vi "WLAN - RxMeasure - Test  - Readwaveform.vi"(0 "VSG Resource Name":refnum<k15>="rio0", 1 "Idle Time/s (With Ack)":dbl, 5 "file path":path, 7 "Power Level(dBm)":dbl, 9 "numPackets":i32=200, 11 "Carrier Frequency(Hz)":dbl, 12 "Path Loss":dbl=1.0) -> ()   [LabVIEW 2010]
uses:
  <instrlib>/niRFSG/niRFSG.llb/niRFSG Ref Clock Sources.ctl
panel:
  in  "stop":bool
  out "LoopTime/ms":u32
  in  "Tab Control":enum32{"Rx_Test Settings", "HW "}(tab)=enum."HW "
  in  "error in (no error)":errorcluster
  out "error out":errorcluster
  # "GET PACKET COUNT (1)"
  # "PACKET STOP"
  # "PACKET START"
  # "GET PACKET COUNT (2)"
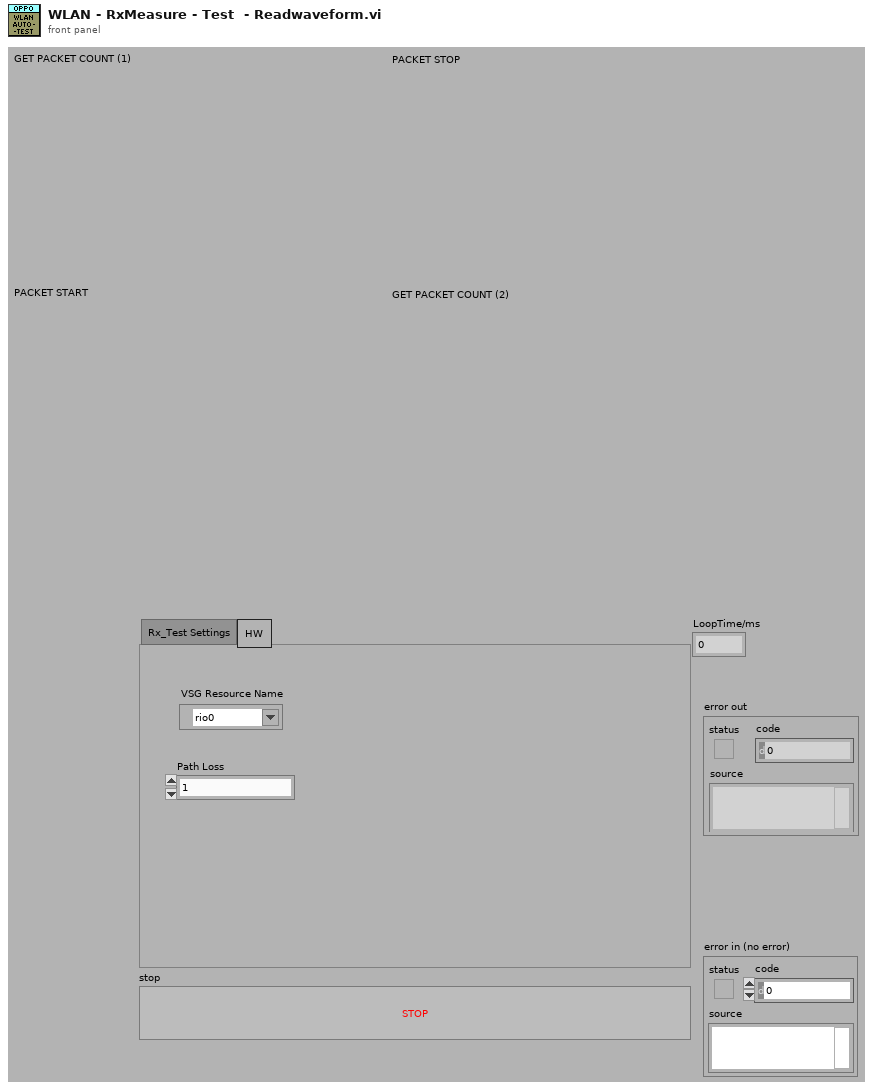
[diagram p1: front panel]
types:
  T1 = typedef "niRFSG Ref Clock Sources.ctl" = string
  T2 = typedef "WLAN - TV - RW - INC - RxTestParameters.ctl" = cluster{"wfm Size in msec":i32, "actual headroom (dB)":dbl, "Size in Samples":i32[], "40M?":bool, "Standard ":i32, "wfm size sec (dbl)":dbl, "dt":dbl, "Channel Bandwidth (Hz)":dbl, "Payload Data Length (bytes)":i32, "80211n PLCP Frame Format":i32, "DSSS Data Rate (Mbps)":i32, "OFDM Data Rate (Mbps)":i32, "MCS Index":i32, "Fc(Hz)":dbl, "#Packets":i32}
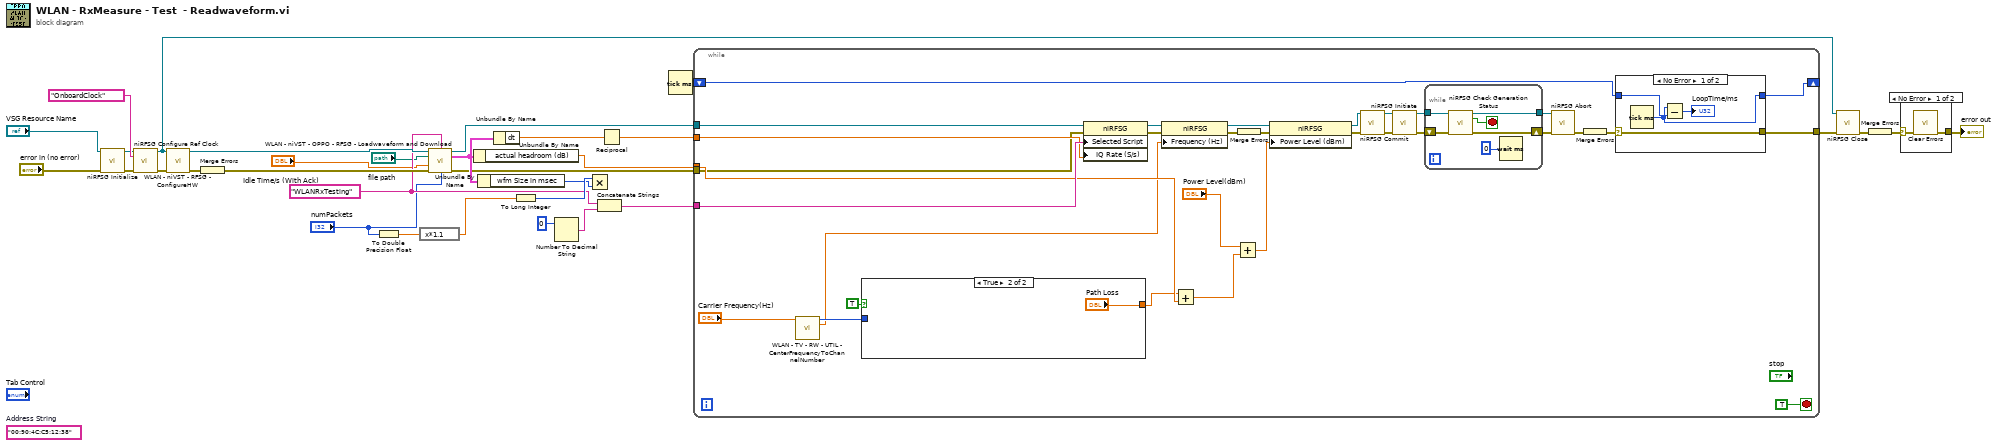
[diagram p0: block diagram]
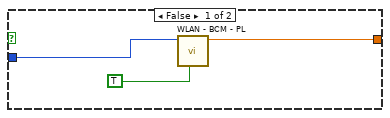
[diagram p2: hidden frame]
diagram:
  w14 = "WLANRxTesting" ("Arb:Selected Script")
  (unwired) "00:90:4C:C5:12:38"  # Address String
  n1 = call <instrlib>:"niRFSG Initialize.vi"("resource name"="VSG Resource Name", "error in"="error in (no error)") -> ("instrument handle"=w20:refnum<k15>, "error out"=w22:errorcluster)  [unwired: 12 in]
  n2 = call <instrlib>:"niRFSG Configure Ref Clock.vi"("instrument handle"=w20, "ref clock source"=T1 "OnboardClock", "error in"=w22) -> ("instrument handle out"=w23:refnum<k15>, "error out"=w21:errorcluster)  [unwired: 11 out]
  n3 = call "WLAN - niVST - RFSG - ConfigureHW.vi"("instrument handle"=w23, "error in"=w21) -> ("instrument handle"=w28:refnum<k15>, "error out"=w27:errorcluster)  [unwired: 12 in]
  n4 = Merge Errors(w27) -> (w15:errorcluster)
  n5 = To Double Precision Float(number="numPackets") -> (double precision float=w18:dbl)
  n6 = expression code="x*1.1"(w18) -> (w19:dbl)
  n7 = call "WLAN - niVST - OPPO - RFSG - Loadwaveform and Download.vi"("instrument handle"=w28, "ScriptName<index>"=w14, "file path"="file path", "Idle Time (With Ack)"="Idle Time/s (With Ack)", "error in"=w15, "numPackets"="numPackets") -> ("instrument handle"=w3:refnum<k15>, "Rx_Test Parameters"=w16:T2, "error out"=w4:errorcluster)  [unwired: 7 in]
  n8 = Unbundle By Name(w16) -> ("actual headroom (dB)"=w8:dbl)
  n9 = Unbundle By Name(w16) -> ("wfm Size in msec"=w9:i32)
  n10 = Unbundle By Name(w16) -> ("dt"=w10:dbl)
  n11 = To Long Integer(number=w19) -> (32bit integer=w17:i32)
  n12 = Number To Decimal String(number=0) -> (decimal integer string=w13:string)  [unwired: 1 in]
  n13 = Multiply(x=w17, y=w9) -> ()  [unwired: 1 out]
  n14 = Concatenate Strings(w14, w13) -> (w12:string)
  n15 = Reciprocal(x=w10) -> (1/x=w11:dbl)
  n16 = Tick Count (ms)() -> (millisecond timer value=w1:u32)
  n17 = while {
    tunnel: [w64] -> w24
    tunnel: w12 -> [w63]
    tunnel: w11 -> [w61]
    tunnel: w8 -> [w56]
    tunnel: w4 -> [w48]
    tunnel: w3 -> [w47]
    shift-right: [w39] -> _
    shift-left: w1 -> [w40]
    stop <- TRUE stop-if-true
    n18 = call "WLAN - TV - RW - UTIL - CenterFrequencyToChannelNumber.vi"("Center Frequency(Hz)"="Carrier Frequency(Hz)") -> ("Coherced Channel Number"=w36:i32, "Coherced Center Frequency (Hz)"=w35:dbl)  [unwired: 13 in]
    n19 = case shown="True" TRUE {
      tunnel: w36 -> [w66 _]
      tunnel: [w65 "Path Loss"] -> w34
      frame False {
        n20 = call "WLAN - BCM - PL.vi"("RX ?"=TRUE, "Channel index"=w66) -> ("PL"=w65:dbl)  [unwired: 9 in]
      }
      frame True {
      }
    }
    n21 = property class="niRFSG"(reference=w47, error in=w48, "Selected Script"=w63, "IQ Rate (S/s)"=w61) -> (reference out=w62:refnum<k15>, error out=w60:errorcluster)
    n22 = property class="niRFSG"(reference=w62, error in=w60, "Frequency (Hz)"=w35) -> (reference out=w59:refnum<k15>, error out=w58:errorcluster)
    n23 = Add(x=w34, y=w56) -> (x+y=w55:dbl)
    n24 = Add(x="Power Level(dBm)", y=w55) -> (x+y=w50:dbl)
    n25 = Merge Errors(w58) -> (w57:errorcluster)
    n26 = property class="niRFSG"(reference=w59, error in=w57, "Power Level (dBm)"=w50) -> (reference out=w53:refnum<k15>, error out=w51:errorcluster)
    n27 = call <instrlib>:"niRFSG Commit.vi"("instrument handle"=w53, "error in"=w51) -> ("instrument handle out"=w52:refnum<k15>, "error out"=w49:errorcluster)  [unwired: 12 in]
    n28 = call <instrlib>:"niRFSG Initiate.vi"("instrument handle"=w52, "error in"=w49) -> ("instrument handle out"=w45:refnum<k15>, "error out"=w43:errorcluster)  [unwired: 12 in]
    n29 = while {
      tunnel: w45 -> [w80]
      tunnel: [w79] -> w44
      shift-right: [w77] -> w42
      shift-left: w43 -> [w76]
      stop <- w78 stop-if-true
      n30 = call <instrlib>:"niRFSG Check Generation Status.vi"("instrument handle"=w80, "error in"=w76) -> ("instrument handle out"=w79:refnum<k15>, "done?"=w78:bool, "error out"=w77:errorcluster)  [unwired: 11 in]
      n31 = Wait (ms)(milliseconds to wait=u32 0) -> ()  [unwired: 1 out]
    }
    n32 = call <instrlib>:"niRFSG Abort.vi"("instrument handle"=w44, "error in"=w42) -> ("error out"=w46:errorcluster)  [unwired: 12 in, 1 out]
    n33 = Merge Errors(w46) -> (w41:errorcluster)
    n34 = case shown="No Error" w41 {
      selector: w41 -> [w69 w73]
      tunnel: w40 -> [w72 w74]
      tunnel: [w71 w74] -> w39
      tunnel: [w69 w73] -> w64
      frame No Error {
        n35 = Tick Count (ms)() -> (millisecond timer value=w71:u32)
        n36 = Subtract(x=w71, y=w72) -> (x-y=→"LoopTime/ms":u32)
      }
      frame Error {
      }
    }
  }
  n37 = call <instrlib>:"niRFSG Close.vi"("instrument handle"=w23, "error in"=w24) -> ("error out"=w31:errorcluster)  [unwired: 13 in]
  n38 = Merge Errors(w31) -> (w25:errorcluster)
  n39 = case shown="No Error" w25 {
    selector: w25 -> [w82 w83]
    tunnel: [w81 w83] -> w29
    frame No Error {
      n40 = call <vilib>:"Clear Errors.vi"("error in (no error)"=w82) -> ("error out"=w81:errorcluster)  [unwired: 6 in]
    }
    frame Error {
    }
  }
  "error out" <- w29
